vi "HexConvertion.vi"(4 "Imaging Protocol":T1, 7 "AOL_Globals":T3={"Imaging Protocol"=enum."AOL Z-Stack", "Number of POI"=0, "Number of Miniscans"=0, "Number of Trials"=0, "Number of Cycles "=0, "# Averaged Frames"=0, "Laser power (%)"=0, "Pockels"=0.0, "Acquisition Length (sec)"=0.0, "Fill time (us)"=0.0, "POI Dwell time (us)"=0.0, "Miniscan Dwell time per pixel (us)"=0.0, "PMT 1"=0.0, "PMT 2"=0.0, "Back Apperture"=200.0, "Frame Size"=0, "Center Frequency"=0.0, "Field of View"=0.0, "DwellTime (us)"=0.0, "Wavelength (nm)"=0.0, "Zoom"=0.0, "AOL Z"=0.0, "AOL Mode"=enum."Raster", "GridXY"=0.0, "GridZ"=0.0, "TriggerPeriod (sec)"=0.0, "Number of Pixels in Miniscan"=0, "Experiment folder path"=path "", "X centre"=0.0, "Y centre"=0.0, "Angle (degrees)"=0.0, "Plane Mode"=0, "Threshold"=[], "Regenerate Chirps"=FALSE, "Rectangle ROI length (pixels)"=0, "Rectangle ROI height (pixels)"=0, "AOD fill"=0, "Samples Wait after Trigger"=0, "StartUp Delay"=0, "Slip Cycle"=163840, "Add Cycle"=FALSE} {"Plane Mode" items=["XY Plane"]; "Frame Size" items=["100X100"=100, "128X128"=128, "200X200"=200, "256X256"=256, "512X512"=512, "1024x1024"=1024, "2048x2048"=2048]; "Back Apperture" format="%#.6g"; "Pockels" format="%#.6g"; "PMT 2" format="%#.6g"; "PMT 1" format="%#.6g"; "Angle (degrees)" format="%#.6g"; "POI Dwell time (us)" format="%#.6g"}, 8 "error in (no error)":errorcluster, 9 "systemVariables":dbl[](array[numeric]), 10 "scanVariables":dbl[][](array[numeric]), 11 "Chirp Parameters":T2) -> (0 "error out":errorcluster, 1 "Interrupted":bool, 3 "HexPackets":string[](array[string]))   [LabVIEW 2013]
uses:
  Typedefs/Controls/AOL_Globals.ctl
  Typedefs/Imaging Protocols enum.ctl
  Typedefs/Frame Size.ctl
  Typedefs/AOL modes.ctl
  Typedefs/Plane Mode.ctl
panel:
  in  "aolAmplitudes":T7={"aod1Amplitude"=210.0, "aod2Amplitude"=150.0, "aod3Amplitude"=190.0, "aod4Amplitude"=150.0}
  # "RE-ENTRANT"
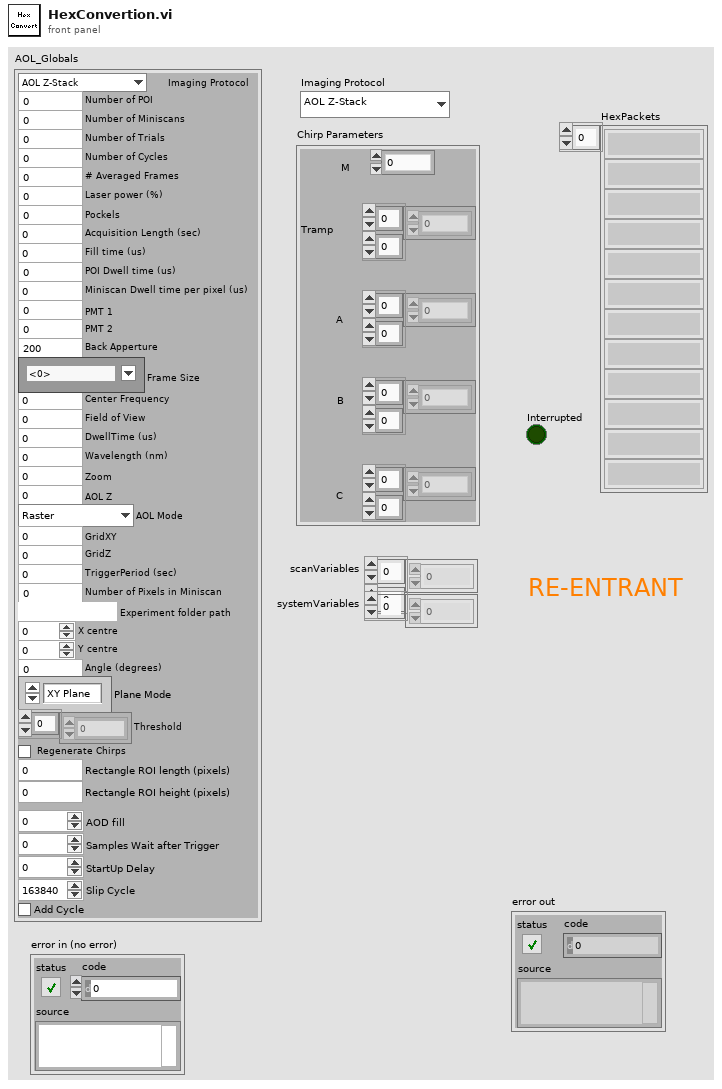
[diagram p1: front panel]
types:
  T1 = typedef "Imaging Protocols enum.ctl" = enum16{"AOL Z-Stack", "Motor Z Stack", "Functional Acquisition", "Single Plane Acquisition", "Volume Acquisition", "Live Imaging", "Live Plane Imaging", "Live Volume Imaging"}
  T2 = cluster{"M ":dbl, "Tramp":dbl[][], "A":dbl[][], "B":dbl[][], "C":dbl[][]}
  T3 = typedef "AOL_Globals.ctl" = cluster{"Imaging Protocol":T1, "Number of POI":u16, "Number of Miniscans":u16, "Number of Trials":u16, "Number of Cycles ":u64, "# Averaged Frames":u16, "Laser power (%)":u8, "Pockels":dbl, "Acquisition Length (sec)":dbl, "Fill time (us)":dbl, "POI Dwell time (us)":dbl, "Miniscan Dwell time per pixel (us)":dbl, "PMT 1":dbl, "PMT 2":dbl, "Back Apperture":dbl, "Frame Size":T4, "Center Frequency":dbl, "Field of View":dbl, "DwellTime (us)":dbl, "Wavelength (nm)":dbl, "Zoom":dbl, "AOL Z":dbl, "AOL Mode":T5, "GridXY":dbl, "GridZ":dbl, "TriggerPeriod (sec)":dbl, "Number of Pixels in Miniscan":u16, "Experiment folder path":path, "X centre":dbl, "Y centre":dbl, "Angle (degrees)":dbl, "Plane Mode":T6, "Threshold":u16[], "Regenerate Chirps":bool, "Rectangle ROI length (pixels)":u16, "Rectangle ROI height (pixels)":u16, "AOD fill":u16, "Samples Wait after Trigger":u16, "StartUp Delay":i32, "Slip Cycle":u32, "Add Cycle":bool}
  T4 = typedef "Frame Size.ctl" = u16
  T5 = typedef "AOL modes.ctl" = enum16{"Raster", "Structural", "Pointing", "Mini Scan", "Alignment"}
  T6 = typedef "Plane Mode.ctl" = u16
  T7 = cluster{"aod1Amplitude":dbl, "aod2Amplitude":dbl, "aod3Amplitude":dbl, "aod4Amplitude":dbl}
  T8 = typedef "Chirp Parameters.ctl" = cluster{"M":dbl, "miniscantime":dbl[], "startfreq":dbl[][], "stopfreq":dbl[][], "nextrampslope":dbl[][], "Hexheader":string, "voxnum":dbl[], "Nvoxdwell":dbl, "miniscanstartX":dbl[], "miniscanstartY":dbl[], "miniscanZ":dbl[], "trigw":dbl, "trigwaodf":dbl, "dn":dbl, "a":dbl[], "A":dbl[][], "B":dbl[][], "Tramp":dbl[][], "C":dbl[][], "Amplitude":dbl[][]}
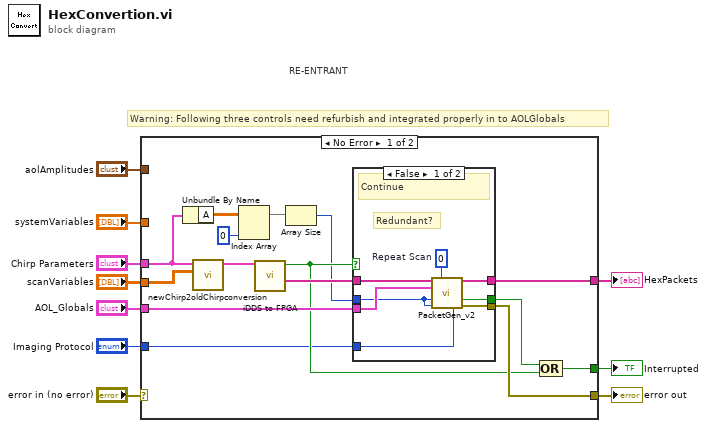
[diagram p0: block diagram]
diagram:
  # "RE-ENTRANT"
  # "Warning: Following three controls need refurbish and integrated properly in to AOLGlobals"
  n1 = case shown="No Error" "error in (no error)" {
    selector: "error in (no error)" -> [_ w34]
    tunnel: [w18 w34] -> w9
    tunnel: "aolAmplitudes" -> [_ _]
    tunnel: "scanVariables" -> [w17 _]
    tunnel: "systemVariables" -> [_ _]
    tunnel: "AOL_Globals" -> [w24 _]
    tunnel: [w23 _] -> w4
    tunnel: "Chirp Parameters" -> [w22 _]
    tunnel: [w14 _] -> w2
    tunnel: "Imaging Protocol" -> [w11 _]
    frame No Error {
      n2 = Unbundle By Name(w22) -> ("A"=w21:dbl[][])
      n3 = call "newChirp2oldChirpconversion.vi"("scanVariables"=w17, "Chirp Parameters"=w22) -> ("ChirpParameters"=w25:T8)  [unwired: 9 in]
      n4 = Index Array(array=w21, index (col)=0 ("disabled index (col)")) -> (element=w20:dbl[])  [unwired: 1 in]
      n5 = call "iDDS to FPGA.vi"("Chirp Parameters"=w25) -> ("HEX Array"=w16:string[], "Interrupted"=w13:bool)  [unwired: 9 in]
      n6 = Array Size(array=w20) -> (size(s)=w12:i32)
      n7 = case shown="False" w13 {
        tunnel: w24 -> [w33 _]
        tunnel: [w32 _] -> w23
        tunnel: w12 -> [w27 _]
        tunnel: [w30 _] -> w18
        tunnel: w16 -> [w29 _]
        tunnel: [w28 _] -> w15
        tunnel: w11 -> [w26 _]
        frame False {
          w31 = 0  # Repeat Scan
          # "Redundant?"
          # "Continue"
          n8 = call "PacketGen_v2.vi"("Hex Array"=w29, "Repeat Scan"=w31, "AOL_Globals"=w33, "Ny"=w27, "Nx"=w27, "Imaging Protocol"=w26) -> ("HexPackets"=w32:string[], "Interrupted"=w28:bool, "error out"=w30:errorcluster)  [unwired: 6 in, 1 out]
        }
        frame True {
          # "Interrupted"
        }
      }
      n9 = Compound Arithmetic op=OR(w15, w13) -> (w14:bool)
    }
    frame Error {
    }
  }
  "error out" <- w9
  "HexPackets" <- w4
  "Interrupted" <- w2
